vi "Write ID.vi"(10 "ID":string, 11 "Simple Actor in":refnum<class "Simple Actor.lvclass">) -> (3 "Simple Actor out":refnum<class "Simple Actor.lvclass">)   [LabVIEW 2017, in "Simple Actor.lvlib" / "Simple Actor.lvclass"]
uses:
  Simple Actor.lvclass
  Simple Actor.lvclass/Simple Actor.ctl
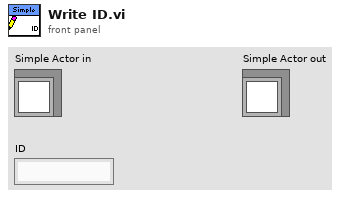
[diagram p1: front panel]
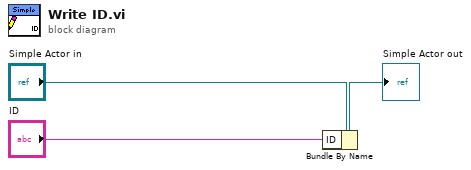
[diagram p0: block diagram]
diagram:
  n1 = Bundle By Name(cluster="Simple Actor in", "ID"="ID") -> (→"Simple Actor out":refnum<class "Simple Actor.lvclass">)
